vi "Car_Speed_R563X.vi"(10 "精度":dbl=0.0625, 11 "车速":u16) -> (3 "报文":T1 {"[7]" format="%02x"; "[6]" format="%02x"; "[5]" format="%02x"; "[4]" format="%02x"; "[3]" format="%02x"; "[2]" format="%02x"; "[1]" format="%02x"; "[0]" format="%02x"})   [LabVIEW 2020]
uses:
  Global_Variable/Global.vi
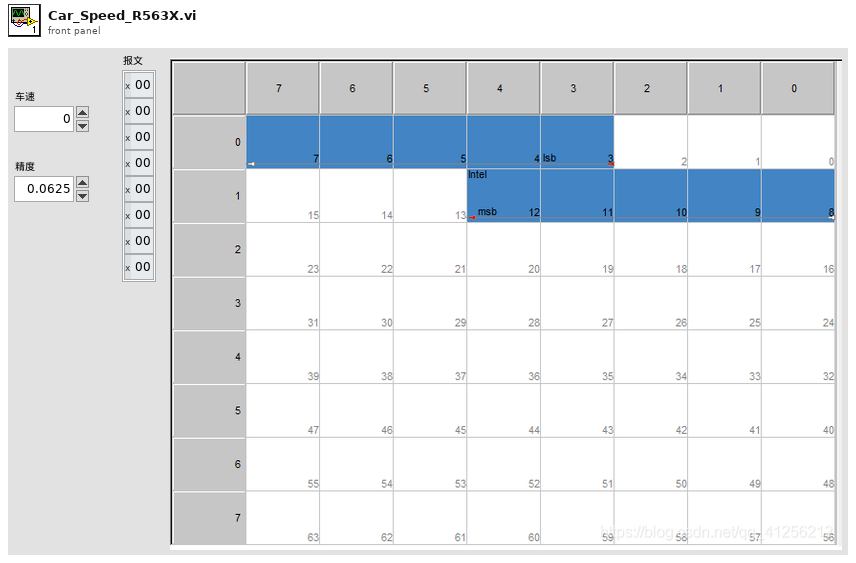
[diagram p1: front panel]
types:
  T1 = cluster{"[0]":u8, "[1]":u8, "[2]":u8, "[3]":u8, "[4]":u8, "[5]":u8, "[6]":u8, "[7]":u8}
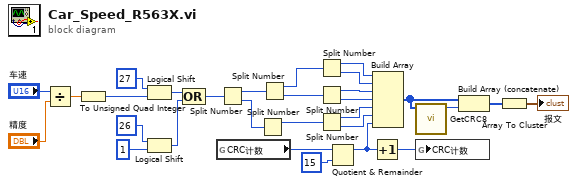
[diagram p0: block diagram]
diagram:
  n1 = Divide(x="车速", y="精度") -> (x/y=w2:dbl)
  n2 = To Unsigned Quad Integer(1:w2) -> (0:w7:u64)
  n3 = Logical Shift(y=i16 27, x=w7) -> (x << y=w18:u64)
  n4 = Logical Shift(y=i16 26, x=u64 1) -> (x << y=w20:u64)
  n5 = Compound Arithmetic op=OR ("复合运算")(w18, w20) -> (w17:u64)
  n6 = global read "Global.vi" "CRC计数"() -> (w4:u8)
  n7 = Split Number(x=w17) -> (hi(x)=w26:u32, lo(x)=w25:u32)
  n8 = Split Number(x=w25) -> (hi(x)=w22:u16)  [unwired: 1 out]
  n9 = Split Number(x=w26) -> (hi(x)=w24:u16, lo(x)=w23:u16)
  n10 = Split Number(x=w24) -> (hi(x)=w16:u8, lo(x)=w15:u8)
  n11 = Split Number(x=w23) -> (hi(x)=w14:u8, lo(x)=w13:u8)
  n12 = Split Number(x=w22) -> (hi(x)=w12:u8, lo(x)=w11:u8)
  n13 = Quotient & Remainder(x=w4, y=u8 15) -> (x-y*floor(x/y)=w5:u8)  [unwired: 1 out]
  n14 = Increment(x=w5) -> (x+1=w3:u8)
  n15 = Build Array(w16, w15, w14, w13, w12, w11, w5) -> (w10:u8[])
  n16 = call "GetCRC8.vi"("xData"=w10) -> ("CRC8"=w9:u8)  [unwired: 9 in, 1 out]
  n17 = global write "Global.vi" "CRC计数"(w3) -> ()
  n18 = Build Array (concatenate)(w10, w9) -> (w8:u8[])
  n19 = Array To Cluster(array=w8) -> (cluster=→"报文":T1)
